vi "Configure DC Volts3.vi"(10 "measurementservice_DMMConfigRequest_Data":T1, 11 "IVI Refnum in":refnum<k15>="DMM" caption="Device Name") -> (0 "error out":errorcluster, 2 "measurementservice_DMMConfigRequest_Data Out":T1)   [LabVIEW 2019, in "HVC3.lvlib" / "HVC3.lvclass"]
uses:
  HVC3 Class/HVC3.lvclass
  HVC3 Class/RPC Messages/measurementservice_DMMConfigRequest/measurementservice_DMMConfigRequest_Data.ctl
  <instrlib>/niDMM/nidmm.llb/niDMM Control Actions.ctl
  <instrlib>/niDMM/nidmm.llb/niDMM Configure Measurement Digits.vi
panel:
  in  "DMM Function Array":i32[](array[numeric])=[1, 2, 3, 4, 5, 101, 1002, 104, 105, 1001, 1005, 1006, 108]
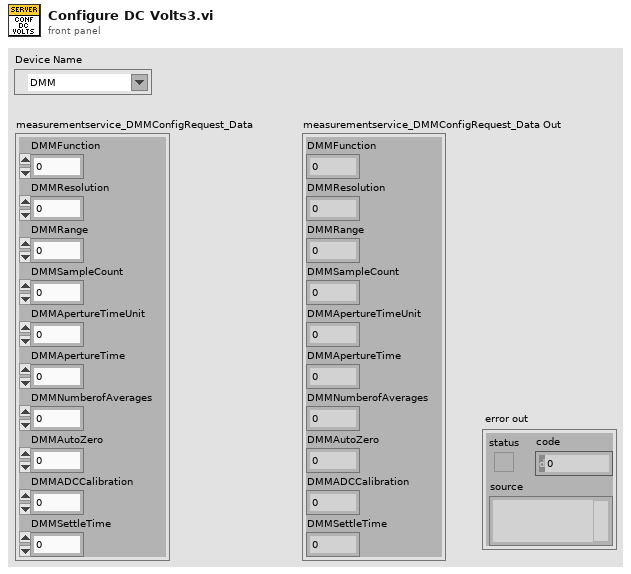
[diagram p1: front panel]
types:
  T1 = typedef "HVC3.lvlib/HVC3.lvclass/measurementservice_DMMConfigRequest_Data.ctl" = cluster{"DMMFunction":i32, "DMMResolution":sgl, "DMMRange":sgl, "DMMSampleCount":i32, "DMMApertureTimeUnit":i32, "DMMApertureTime":sgl, "DMMNumberofAverages":i32, "DMMAutoZero":i32, "DMMADCCalibration":i32, "DMMSettleTime":sgl}
  T2 = typedef "niDMM Control Actions.ctl" = i32
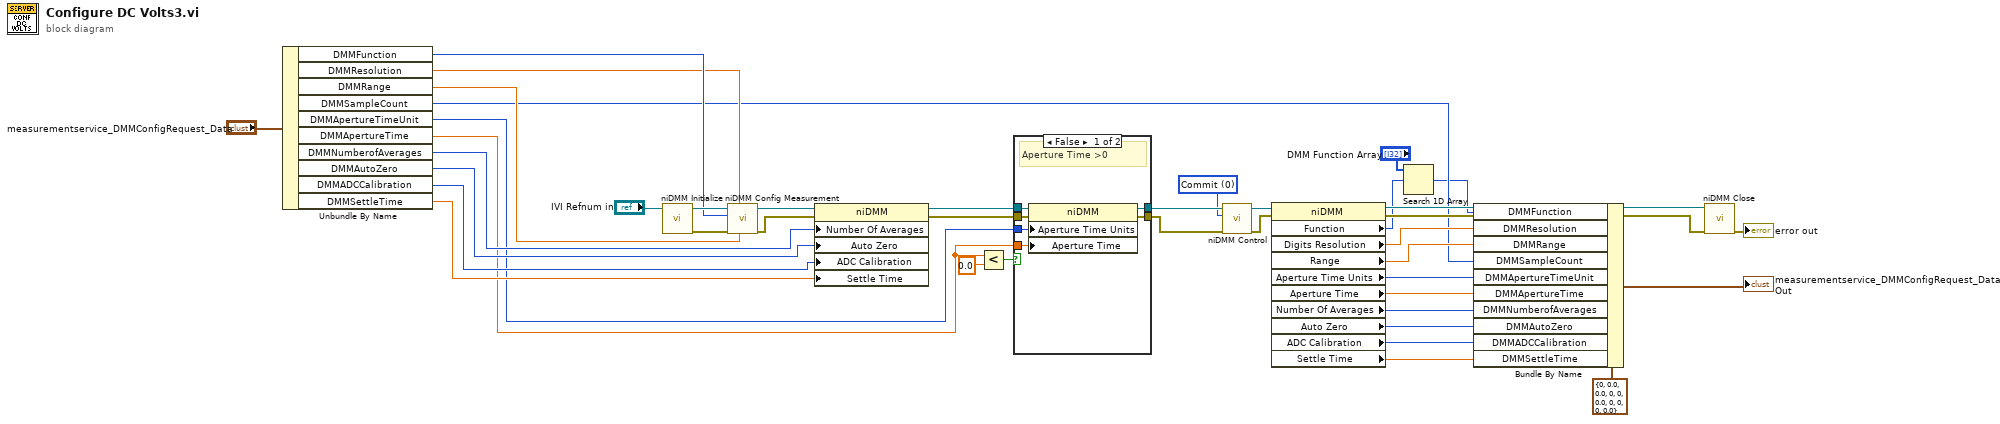
[diagram p0: block diagram]
diagram:
  w19 = T2 0 items=["Commit"] ("Control Action")
  n1 = Unbundle By Name("measurementservice_DMMConfigRequest_Data") -> ("DMMFunction"=w37:i32, "DMMResolution"=w36:sgl, "DMMRange"=w35:sgl, "DMMSampleCount"=w4:i32, "DMMApertureTimeUnit"=w24:i32, "DMMApertureTime"=w23:sgl, "DMMNumberofAverages"=w32:i32, "DMMAutoZero"=w31:i32, "DMMADCCalibration"=w30:i32, "DMMSettleTime"=w29:sgl)
  n2 = call <instrlib>:"niDMM Initialize.vi"("Instrument Descriptor"="IVI Refnum in") -> ("error out"=w39:errorcluster, "instrument handle out"=w40:refnum<k15>)  [unwired: 9 in]
  n3 = call-poly <instrlib>:"niDMM Config Measurement.vi"("Range"=w35, "Resolution in Digits"=w36, "error in (no error)"=w39, "Function"=w37, "instrument handle"=w40) -> ("error out"=w33:errorcluster, "instrument handle out"=w34:refnum<k15>)  [unwired: 5 in]
  n4 = property class="niDMM"(reference=w34, error in=w33, "Number Of Averages"=w32, "Auto Zero"=w31, "ADC Calibration"=w30, "Settle Time"=w29) -> (reference out=w28:refnum<k15>, error out=w27:errorcluster)
  n5 = Less?(x=w23, y=0.0 ("Configuration:Advanced:Aperture Time")) -> (x < y?=w25:bool)
  n6 = case shown="False" w25 {
    tunnel: w28 -> [w47 w49]
    tunnel: w27 -> [w46 w48]
    tunnel: [w45 w49] -> w21
    tunnel: [w44 w48] -> w20
    tunnel: w24 -> [w43 _]
    tunnel: w23 -> [w42 _]
    frame False {
      # "Aperture Time >0"
      n7 = property class="niDMM"(reference=w47, error in=w46, "Aperture Time Units"=w43, "Aperture Time"=w42) -> (reference out=w45:refnum<k15>, error out=w44:errorcluster)
    }
    frame True {
      # "Aperture Time <0"
    }
  }
  n8 = call <instrlib>:"niDMM Control.vi"("error in (no error)"=w20, "Control Action"=w19, "instrument handle"=w21) -> ("error out"=w17:errorcluster, "instrument handle out"=w18:refnum<k15>)  [unwired: 7 in]
  n9 = property class="niDMM"(reference=w18, error in=w17) -> (reference out=w16:refnum<k15>, error out=w15:errorcluster, "Function"=w2:i32, "Digits Resolution"=w6:dbl, "Range"=w7:dbl, "Aperture Time Units"=w8:i32, "Aperture Time"=w9:dbl, "Number Of Averages"=w10:i32, "Auto Zero"=w11:i32, "ADC Calibration"=w12:i32, "Settle Time"=w13:dbl)
  n10 = Search 1D Array(1D array="DMM Function Array", element=w2) -> (index of element=w1:i32)  [unwired: 1 in]
  n11 = Bundle By Name(cluster=T1 {"DMMFunction"=0, "DMMResolution"=0.0, "DMMRange"=0.0, "DMMSampleCount"=0, "DMMApertureTimeUnit"=0, "DMMApertureTime"=0.0, "DMMNumberofAverages"=0, "DMMAutoZero"=0, "DMMADCCalibration"=0, "DMMSettleTime"=0.0} ("measurementservice_DMMConfigRequest_Data Out"), "DMMFunction"=w1, "DMMResolution"=w6, "DMMRange"=w7, "DMMSampleCount"=w4, "DMMApertureTimeUnit"=w8, "DMMApertureTime"=w9, "DMMNumberofAverages"=w10, "DMMAutoZero"=w11, "DMMADCCalibration"=w12, "DMMSettleTime"=w13) -> (→"measurementservice_DMMConfigRequest_Data Out":T1)
  n12 = call <instrlib>:"niDMM Close.vi"("error in (no error)"=w15, "instrument handle"=w16) -> ("error out"=→"error out":errorcluster)  [unwired: 9 in]
